vi "Extract Rectangle Values(SubVI).vi"(11 "Particle Measurements (Pixels)":dbl[][](array[numeric])) -> (3 "Cluster":T1)   [LabVIEW 2014]
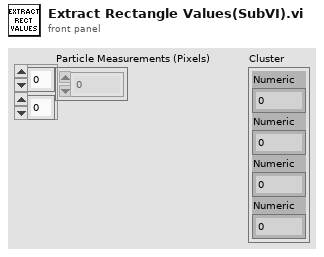
[diagram p1: front panel]
types:
  T1 = cluster{"Numeric":dbl, "Numeric":dbl, "Numeric":dbl, "Numeric":dbl}
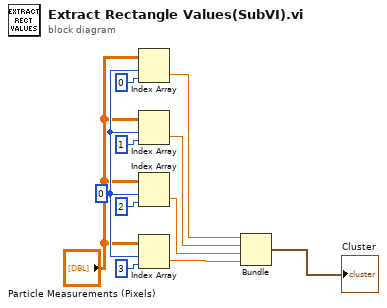
[diagram p0: block diagram]
diagram:
  w2 = 0 ("index (row)")
  n1 = Index Array(array="Particle Measurements (Pixels)", index (row)=w2, index (col)=0 ("disabled index (col)")) -> (element=w7:dbl)
  n2 = Index Array(array="Particle Measurements (Pixels)", index (row)=w2, index (col)=1 ("disabled index (col)")) -> (element=w8:dbl)
  n3 = Index Array(array="Particle Measurements (Pixels)", index (row)=w2, index (col)=2 ("disabled index (col)")) -> (element=w9:dbl)
  n4 = Index Array(array="Particle Measurements (Pixels)", index (row)=w2, index (col)=3 ("disabled index (col)")) -> (element=w10:dbl)
  n5 = Bundle("Numeric"=w7, "Numeric"=w8, "Numeric"=w9, "Numeric"=w10) -> (→"Cluster":T1)  [unwired: 1 in]
